vi "Autonomous Independent.vi"() -> ()   [LabVIEW 2017]
doc: "This VI is called when autonomous begins, and will automatically be terminated when autonomous ends. You can carry out timed or sensor driven robot movement independently without needing to return to the caller."
uses:
  <vilib>/Rock Robotics/WPI/Utilities/WPI_GetSetVariantRefNum.vi
  <vilib>/Rock Robotics/Network Tables/NT Read String.vi
  Robot Global Data.vi
  <vilib>/Rock Robotics/WPI/Solenoid/Deprecated/WPI_SolenoidSetBool.vi
  <vilib>/Rock Robotics/Network Tables/NT Write Numeric Array.vi
panel:
  in  "Array of robot movements 3":T1(array[cluster])=[{"Joystick Left"=-1.0, "Delay (sec)"=3.0, "Joystick Right"=-1.0, "Extend"=FALSE, "Open"=FALSE, " Close"=FALSE, " Retract"=FALSE, "Left Distance"=60.0, "Right Distance"=60.0}, {"Joystick Left"=0.0, "Delay (sec)"=0.0, "Joystick Right"=0.0, "Extend"=FALSE, "Open"=FALSE, " Close"=FALSE, " Retract"=FALSE, "Left Distance"=0.0, "Right Distance"=0.0}]
  # "Be sure to right-click and choose Data Operations>>Make Current Value default if you want to save the array values with the VI"
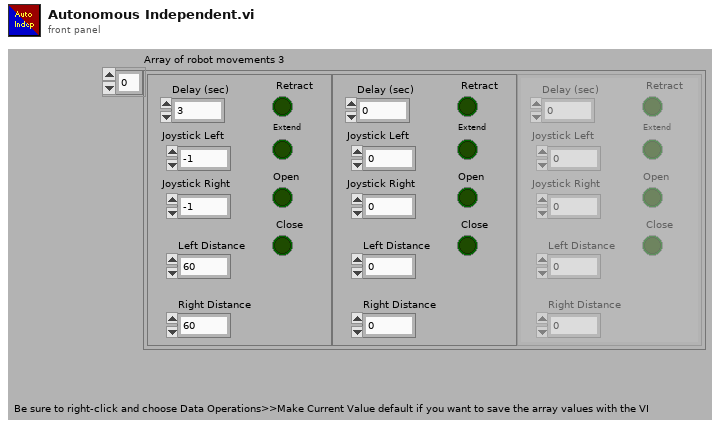
[diagram p1: front panel]
types:
  T1 = cluster{"Joystick Left":dbl, "Delay (sec)":dbl, "Joystick Right":dbl, "Extend":bool, "Open":bool, " Close":bool, " Retract":bool, "Left Distance":dbl, "Right Distance":dbl}[]
  T2 = typedef "WPI_JoystickDevRef.ctl" = cluster{"Device":T3}
  T3 = typedef "WPI_JoystickDeviceEnum.ctl" = enum16{"USB 0", "USB 1", "USB 2", "USB 3", "USB 4", "USB 5"}
  T4 = typedef "WPI_RobotDriveDevRef.ctl" = cluster{"DevStatus":errorcluster, "Motors[]":T5[], "Square Inputs":bool, "Max Output":dbl}
  T5 = typedef "WPI_MotorControlDeviceRef.ctl" = cluster{"DeviceStatus":errorcluster, "Type":T6, "PWM":cluster{"PWM Channel":T7, "DeadBand":T8}, "CAN":cluster{"Device Number":u8, "SetOutput VI Ref":variant, "GetOutput VI Ref":variant, "Enable VI Ref":variant, "Disable VI Ref":variant, "Data":variant}, "Invert":bool, "DIO PWM":cluster{"PWM \"Enable\" Channel":T7, "DIOChannel":T9, "PWM Rate":dbl}}
  T6 = typedef "WPI_MotorControlType.ctl" = enum16{"PWM", "CAN", "DIO PWM"}
  T7 = typedef "FPGA_DIOPWMChannel.ctl" = enum8{"PWM 0", "PWM 1", "PWM 2", "PWM 3", "PWM 4", "PWM 5", "PWM 6", "PWM 7", "PWM 8", "PWM 9", "PWM MXP 0", "PWM MXP 1", "PWM MXP 2", "PWM MXP 3", "PWM MXP 4", "PWM MXP 5", "PWM MXP 6", "PWM MXP 7", "PWM MXP 8", "PWM MXP 9", "Invalid"}
  T8 = typedef "WPI_PWMDeadband.ctl" = cluster{"Name":string, "maxPositivePwm":i32, "minPositivePwm":i32, "centerPwm":i32, "maxNegativePwm":i32, "minNegativePwm":i32, "angularRange":u16}
  T9 = typedef "FPGA_DIOChannel.ctl" = enum8{"DIO 0", "DIO 1", "DIO 2", "DIO 3", "DIO 4", "DIO 5", "DIO 6", "DIO 7", "DIO 8", "DIO 9", "DIO MXP 0", "DIO MXP 1", "DIO MXP 2", "DIO MXP 3", "DIO MXP 4", "DIO MXP 5", "DIO MXP 6", "DIO MXP 7", "DIO MXP 8", "DIO MXP 9", "DIO MXP 10", "DIO MXP 11", "DIO MXP 12", "DIO MXP 13", "DIO MXP 14", "DIO MXP 15", "SPI Port CS1", "SPI Port CS2", "SPI Port CS3", "SPI Port MISO", "SPI Port MOSI", "Invalid"}
  T10 = typedef "WPI_SolenoidDevRef.ctl" = cluster{"DevStatus":errorcluster, "Pneumatics Control Module":u8, "Forward Solenoid Channel":T11, "Reverse Solenoid Channel":T11}
  T11 = typedef "WPI_SolenoidChannel.ctl" = enum8{"Solenoid 0", "Solenoid 1", "Solenoid 2", "Solenoid 3", "Solenoid 4", "Solenoid 5", "Solenoid 6", "Solenoid 7", "Invalid"}
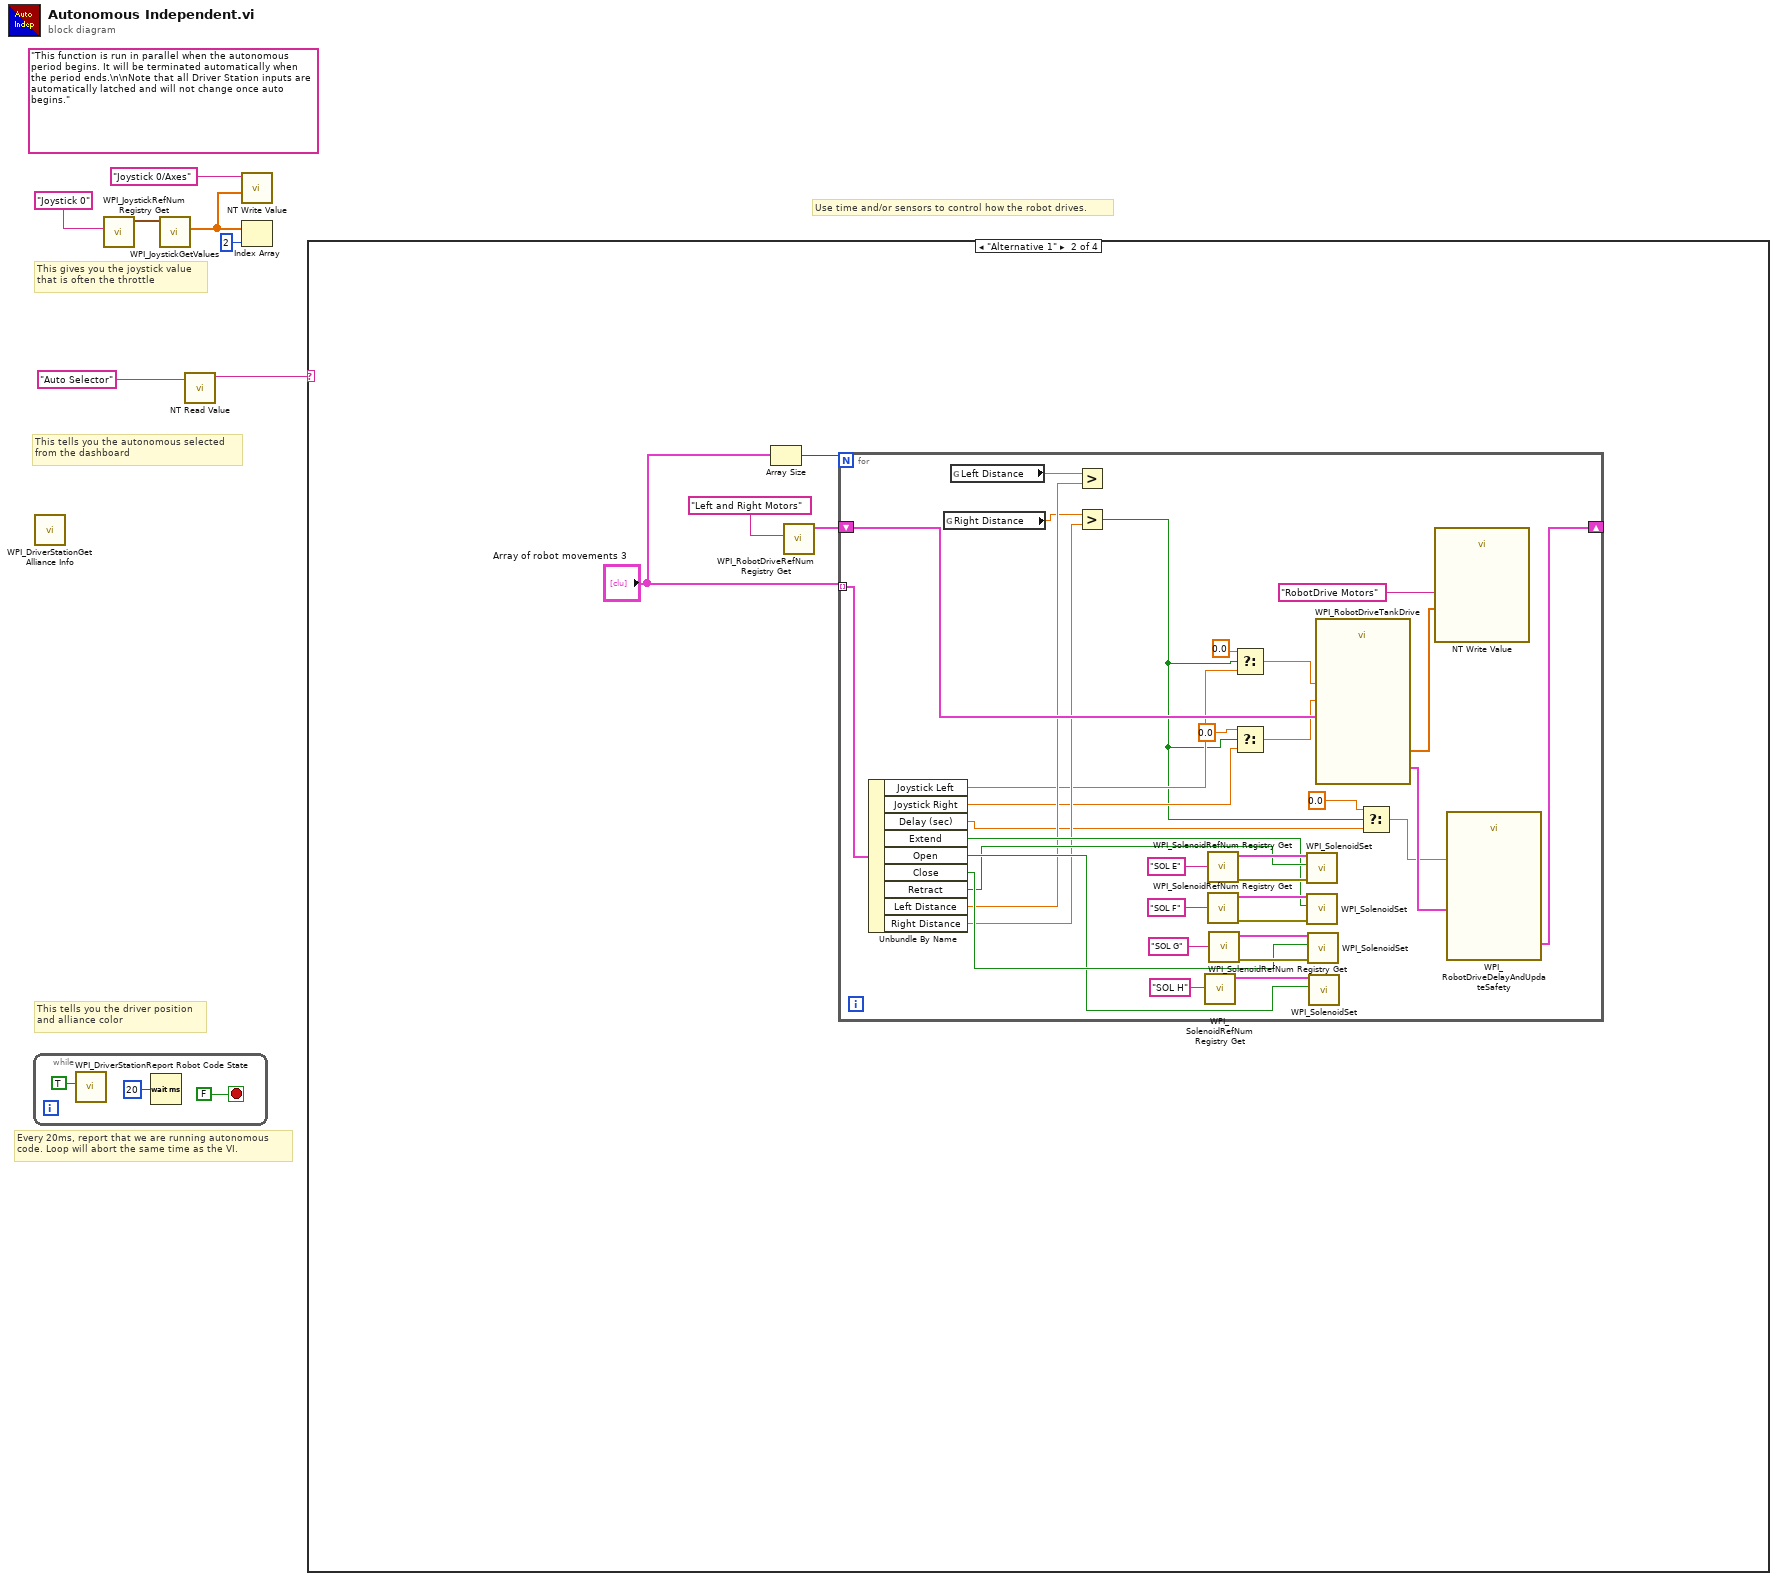
[diagram p0: block diagram]
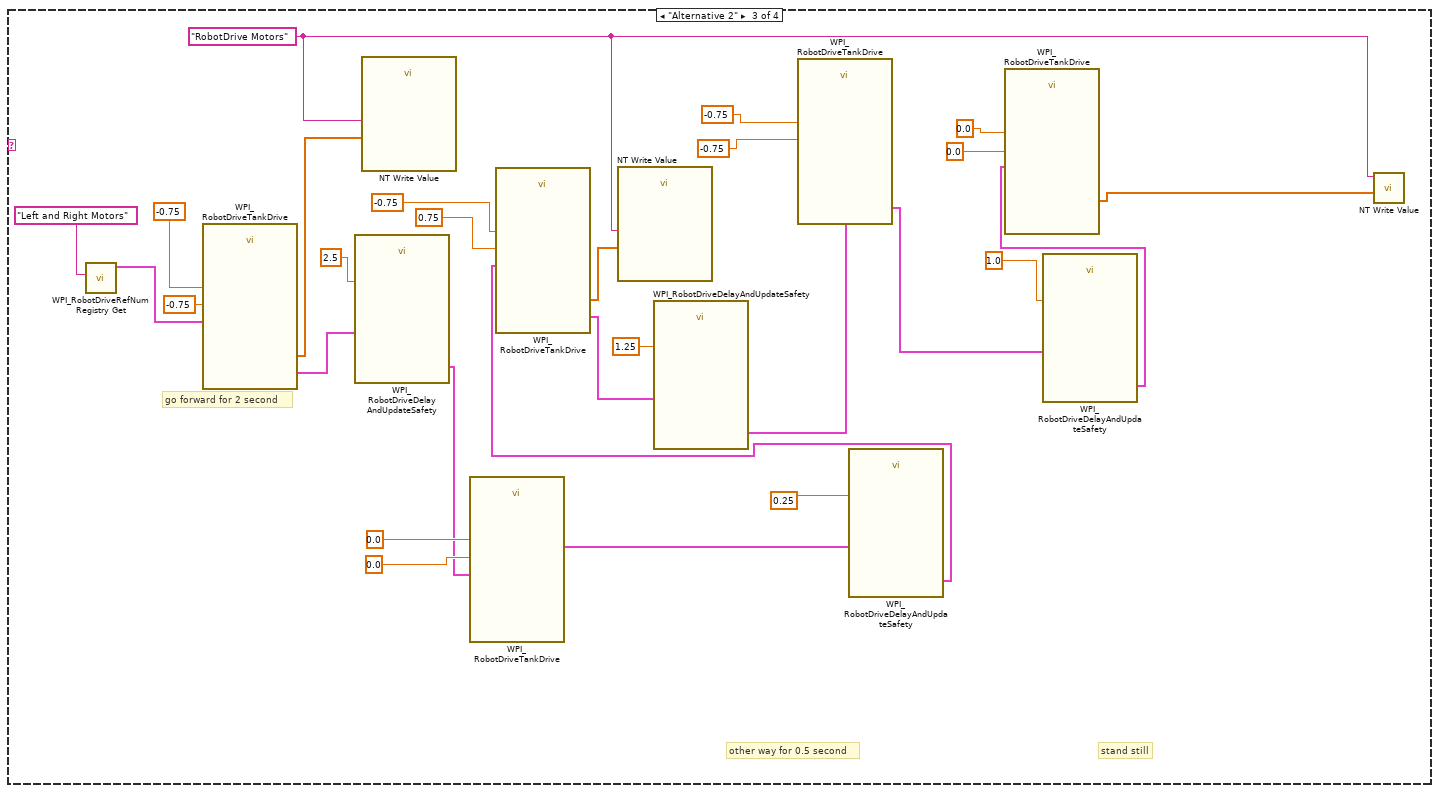
[diagram p3: hidden frame]
diagram:
  (unwired) "This function is run in parallel when the autonomous period begins. It will be terminated automatically when the period ends.\n\nNote that all Driver Station inputs are automatically latched and will not change once auto begins."
  # "This tells you the autonomous selected\nfrom the dashboard"
  # "Every 20ms, report that we are running autonomous\ncode. Loop will abort the same time as the VI."
  # "This gives you the joystick value\nthat is often the throttle"
  # "Use time and/or sensors to control how the robot drives."
  # "This tells you the driver position\nand alliance color"
  n1 = while {
    stop <- FALSE stop-if-true
    n2 = call <vilib>:"WPI_DriverStationReport Robot Code State.vi"("Autonomous"=TRUE) -> ()  [unwired: 10 in, 1 out]
    n3 = Wait (ms)(milliseconds to wait=u32 20) -> ()  [unwired: 1 out]
  }
  n4 = call <vilib>:"WPI_DriverStationGet Alliance Info.vi"() -> ()  [unwired: 12 out]
  n5 = call <vilib>:"WPI_JoystickRefNum Registry Get.vi"("refnum name"="Joystick 0") -> ("JoystickDevRef"=w6:T2)  [unwired: 1 in, 9 out]
  n6 = call <vilib>:"WPI_JoystickGetValues.vi"("JoystickDevRef"=w6) -> ("Axes"=w2:dbl[])  [unwired: 6 in, 4 out]
  n7 = call-poly <vilib>:"NT Read Value.vi"("Name"="Auto Selector") -> ("String"=w3:string)  [unwired: 9 in, 1 out]
  n8 = call-poly <vilib>:"NT Write Value.vi"("Numeric Array"=w2, "Name"="Joystick 0/Axes") -> ()  [unwired: 9 in, 1 out]
  n9 = Index Array(array=w2, index=2) -> ()  [unwired: 1 out]
  n10 = case shown="\"Alternative 1\"" w3 {
    frame Default {
      # "You can put your main auto here, or you can right-click on the case and make any\nother frame be the default case."
      # "This is the frame that will execute if no selection is made, or if it is not recognized"
    }
    frame "Alternative 1" {
      n11 = Array Size(array="Array of robot movements 3") -> (size(s)=w12:i32)
      n12 = call <vilib>:"WPI_RobotDriveRefNum Registry Get.vi"("refnum name"="Left and Right Motors") -> ("RobotDriveDevRef"=w13:T4)  [unwired: 1 in, 9 out]
      n13 = for {
        N: w12 -> [_]
        shift-right: [w47] -> _
        shift-left: w13 -> [w48]
        tunnel: "Array of robot movements 3" -> [w46] mode=indexing
        n14 = Unbundle By Name(w46) -> ("Joystick Left"=w17:dbl, "Joystick Right"=w19:dbl, "Delay (sec)"=w22:dbl, "Extend"=w29:bool, "Open"=w31:bool, "Close"=w32:bool, "Retract"=w30:bool, "Left Distance"=w27:dbl, "Right Distance"=w26:dbl)
        n15 = global read "Robot Global Data.vi" "Right Distance"() -> (w24:dbl)
        n16 = global read "Robot Global Data.vi" "Left Distance"() -> (w28:dbl)
        n17 = Greater?(x=w28, y=w27) -> ()  [unwired: 1 out]
        n18 = Greater?(x=w24, y=w26) -> (0:w15:bool)
        n19 = call <vilib>:"WPI_SolenoidRefNum Registry Get.vi"("refnum name"="SOL H") -> ("SolenoidDevRef"=w43:T10)  [unwired: 9 in, 1 out]
        n20 = call <vilib>:"WPI_SolenoidRefNum Registry Get.vi"("refnum name"="SOL E") -> ("error out"=w38:errorcluster, "SolenoidDevRef"=w37:T10)  [unwired: 9 in]
        n21 = call <vilib>:"WPI_SolenoidRefNum Registry Get.vi"("refnum name"="SOL F") -> ("error out"=w40:errorcluster, "SolenoidDevRef"=w39:T10)  [unwired: 9 in]
        n22 = call <vilib>:"WPI_SolenoidRefNum Registry Get.vi"("refnum name"="SOL G") -> ("error out"=w42:errorcluster, "SolenoidDevRef"=w41:T10)  [unwired: 9 in]
        n23 = Select(t=0.0, s=w15, f=w17) -> (s? t:f=w16:dbl)
        n24 = Select(t=0.0, s=w15, f=w19) -> (s? t:f=w18:dbl)
        n25 = call-poly <vilib>:"WPI_SolenoidSet.vi"("error in (no error)"=w38, "Value"=w30, "SolenoidDevRef"=w37) -> ()  [unwired: 7 in, 2 out]
        n26 = call-poly <vilib>:"WPI_SolenoidSet.vi"("error in (no error)"=w40, "Value"=w29, "SolenoidDevRef"=w39) -> ()  [unwired: 7 in, 2 out]
        n27 = call-poly <vilib>:"WPI_SolenoidSet.vi"("error in (no error)"=w42, "Value"=w32, "SolenoidDevRef"=w41) -> ()  [unwired: 7 in, 2 out]
        n28 = call-poly <vilib>:"WPI_SolenoidSet.vi"("Value"=w31, "SolenoidDevRef"=w43) -> ()  [unwired: 8 in, 2 out]
        n29 = call <vilib>:"WPI_RobotDriveTankDrive.vi"("Right axis value"=w18, "Left axis value"=w16, "RobotDriveDevRef"=w48) -> ("Motor Values"=w44:dbl[], "RobotDriveDevRef"=w49:T4)  [unwired: 6 in, 1 out]
        n30 = Select(t=0.0, s=w15, f=w22) -> (s? t:f=w25:dbl)
        n31 = call-poly <vilib>:"NT Write Value.vi"("Numeric Array"=w44, "Name"="RobotDrive Motors") -> ()  [unwired: 9 in, 1 out]
        n32 = call <vilib>:"WPI_RobotDriveDelayAndUpdateSafety.vi"("Delay (s)"=w25, "RobotDriveDevRef"=w49) -> ("RobotDriveDevRef 2"=w47:T4)  [unwired: 8 in, 1 out]
      }
    }
    frame "Alternative 2" {
      w63 = "RobotDrive Motors" ("Name")
      # "stand still"
      # "other way for 0.5 second"
      # "go forward for 2 second"
      n33 = call <vilib>:"WPI_RobotDriveRefNum Registry Get.vi"("refnum name"="Left and Right Motors") -> ("RobotDriveDevRef"=w77:T4)  [unwired: 1 in, 9 out]
      n34 = call <vilib>:"WPI_RobotDriveTankDrive.vi"("Right axis value"=-0.75 ("X axis value"), "Left axis value"=-0.75 ("X axis value"), "RobotDriveDevRef"=w77) -> ("Motor Values"=w62:dbl[], "RobotDriveDevRef"=w71:T4)  [unwired: 6 in, 1 out]
      n35 = call <vilib>:"WPI_RobotDriveDelayAndUpdateSafety.vi"("Delay (s)"=2.5, "RobotDriveDevRef"=w71) -> ("RobotDriveDevRef 2"=w53:T4)  [unwired: 8 in, 1 out]
      n36 = call-poly <vilib>:"NT Write Value.vi"("Numeric Array"=w62, "Name"=w63) -> ()  [unwired: 9 in, 1 out]
      n37 = call <vilib>:"WPI_RobotDriveTankDrive.vi"("Right axis value"=0.0, "Left axis value"=0.0, "RobotDriveDevRef"=w53) -> ("RobotDriveDevRef"=w51:T4)  [unwired: 6 in, 2 out]
      n38 = call <vilib>:"WPI_RobotDriveDelayAndUpdateSafety.vi"("Delay (s)"=0.25, "RobotDriveDevRef"=w51) -> ("RobotDriveDevRef 2"=w50:T4)  [unwired: 8 in, 1 out]
      n39 = call <vilib>:"WPI_RobotDriveTankDrive.vi"("Right axis value"=0.75 ("X axis value"), "Left axis value"=-0.75 ("X axis value"), "RobotDriveDevRef"=w50) -> ("Motor Values"=w64:dbl[], "RobotDriveDevRef"=w72:T4)  [unwired: 6 in, 1 out]
      n40 = call-poly <vilib>:"NT Write Value.vi"("Numeric Array"=w64, "Name"=w63) -> ()  [unwired: 9 in, 1 out]
      n41 = call <vilib>:"WPI_RobotDriveDelayAndUpdateSafety.vi"("Delay (s)"=1.25, "RobotDriveDevRef"=w72) -> ("RobotDriveDevRef 2"=w73:T4)  [unwired: 8 in, 1 out]
      n42 = call <vilib>:"WPI_RobotDriveTankDrive.vi"("Right axis value"=-0.75 ("X axis value"), "Left axis value"=-0.75 ("X axis value"), "RobotDriveDevRef"=w73) -> ("RobotDriveDevRef"=w60:T4)  [unwired: 6 in, 2 out]
      n43 = call <vilib>:"WPI_RobotDriveDelayAndUpdateSafety.vi"("Delay (s)"=1.0, "RobotDriveDevRef"=w60) -> ("RobotDriveDevRef 2"=w59:T4)  [unwired: 8 in, 1 out]
      n44 = call <vilib>:"WPI_RobotDriveTankDrive.vi"("Right axis value"=0.0, "Left axis value"=0.0, "RobotDriveDevRef"=w59) -> ("Motor Values"=w58:dbl[])  [unwired: 6 in, 2 out]
      n45 = call-poly <vilib>:"NT Write Value.vi"("Numeric Array"=w58, "Name"=w63) -> ()  [unwired: 9 in, 1 out]
    }
    frame "Your Turn" {
    }
  }
